vi "Get - Window Name Index.vi"(0 "reference in":refnum<class "SPWB.lvclass">, 5 "error in (no error)":errorcluster) -> (13 "Window Name Index":string, 14 "reference out":refnum<class "SPWB.lvclass">, 19 "error out":errorcluster)   [LabVIEW 2020, in "SPWB.lvclass"]
uses:
  SPWB.lvclass
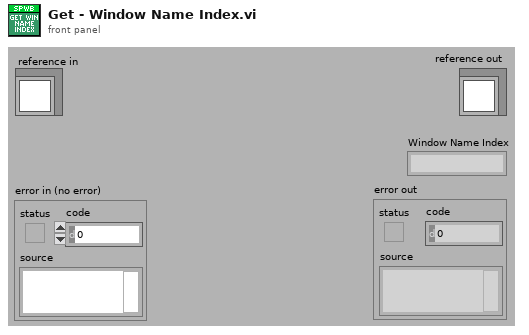
[diagram p1: front panel]
types:
  T1 = typedef "SPWB.lvclass/ObjectAttributes.ctl" = cluster{"Window Name Index":string, "Data":refnum<class "GSwFormDSP.lvclass">, "Registration":refnum<class "Registration.lvclass">, "TFA User Control Refs ":T2}
  T2 = typedef "SPWB.lvclass/TFA - User Control References.ctl" = cluster{"STFT Graph":refnum<vi>, "Time Section":refnum<vi>, "Frequency Section":refnum<vi>}
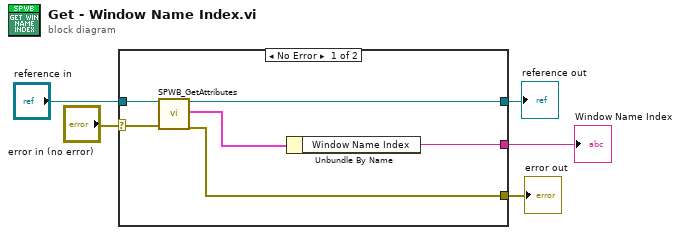
[diagram p0: block diagram]
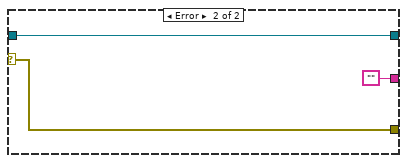
[diagram p2: hidden frame]
diagram:
  n1 = case shown="No Error" "error in (no error)" {
    selector: "error in (no error)" -> [w11 w14]
    tunnel: [w10 w14] -> w4
    tunnel: [w9 w13] -> w2
    tunnel: "reference in" -> [w7 w13]
    tunnel: [w6 ""] -> w1
    frame No Error {
      n2 = call "SPWB_GetAttributes.vi"("reference in"=w7, "error in (no error)"=w11) -> ("reference out"=w9:refnum<class "SPWB.lvclass">, "attributes"=w8:T1, "error out"=w10:errorcluster)  [unwired: 14 in, 1 out]
      n3 = Unbundle By Name(w8) -> ("Window Name Index"=w6:string)
    }
    frame Error {
    }
  }
  "error out" <- w4
  "reference out" <- w2
  "Window Name Index" <- w1
